vi "niRFUtil MT UTIL Check Flush State.vi"(0 "reset?":bool, 5 "flush buffers? (F)":bool, 11 "error in (no error)":errorcluster) -> (15 "error out":errorcluster)   [LabVIEW 2015, in "niRFUtil.lvlib"]
uses:
  niRFUtil.lvlib
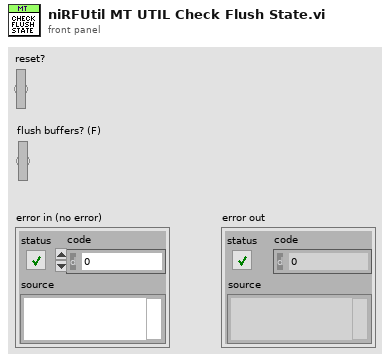
[diagram p1: front panel]
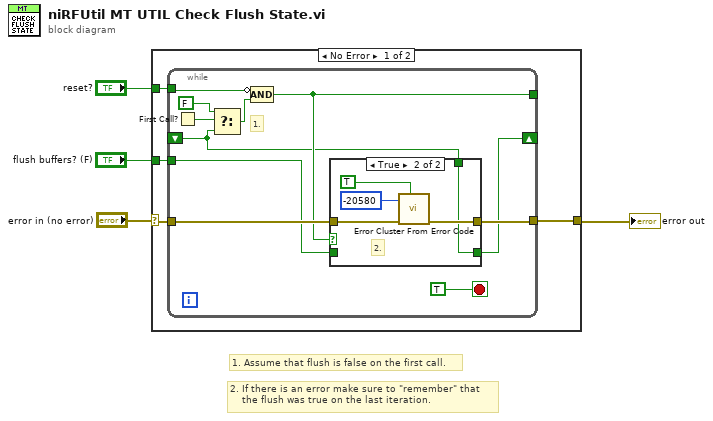
[diagram p0: block diagram]
diagram:
  # "2. If there is an error make sure to \"remember\" that\n    the flush was true on the last iteration."
  # "1. Assume that flush is false on the first call."
  n1 = case shown="No Error" "error in (no error)" {
    selector: "error in (no error)" -> [w5 w27]
    tunnel: "flush buffers? (F)" -> [w8 _]
    tunnel: "reset?" -> [w7 _]
    tunnel: [w6 w27] -> w1
    frame No Error {
      n2 = while {
        tunnel: w8 -> [w11]
        shift-right: [w10] -> _
        shift-left: _ -> [w9]
        tunnel: w7 -> [w19]
        tunnel: [w12] -> _
        tunnel: [w14] -> w6
        tunnel: w5 -> [w13]
        stop <- TRUE stop-if-true
        # "1."
        n3 = First Call?() -> (First Call?: T/F=w17:bool)
        n4 = Select(t=FALSE, s=w17, f=w9) -> (s? t:f=w15:bool)
        n5 = Compound Arithmetic op=AND(invert w19, w15) -> (w12:bool)
        n6 = case shown="True" w12 {
          tunnel: w13 -> [w21 w24]
          tunnel: [w21 w23] -> w14
          tunnel: w11 -> [w20 _]
          tunnel: [w20 w22] -> w10
          tunnel: w9 -> [_ w22]
          frame False {
          }
          frame True {
            # "2."
            n7 = call <vilib>:"Error Cluster From Error Code.vi"("show call chain? (False)"=TRUE, "error in (no error)"=w24, "error code (0)"=-20580) -> ("error out"=w23:errorcluster)  [unwired: 6 out]
          }
        }
      }
    }
    frame Error {
    }
  }
  "error out" <- w1
